vi "Problem2.1.vi"() -> ()   [LabVIEW 2019]
panel:
  out "Time in Seconds":u32
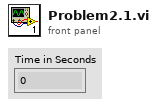
[diagram p1: front panel]
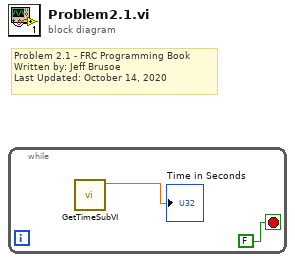
[diagram p0: block diagram]
diagram:
  # "Problem 2.1 - FRC Programming Book\nWritten by: Jeff Brusoe\nLast Updated: October 14, 2020"
  n1 = while {
    stop <- FALSE stop-if-true
    n2 = call "GetTimeSubVI.vi"() -> ("Seconds"=→"Time in Seconds":dbl)  [unwired: 11 in]
  }
